vi "MAIN GENERA FILES STRINGHE.vi"(11 "This VI (main)":refnum<vi>) -> ()   [LabVIEW 2019]
uses:
  <vilib>/Utility/file.llb/Write Delimited Spreadsheet (string).vi
panel:
  out "Costanti":string[][](array[string])
  out "PageLabels":string[][](array[string])
  out "Strings[4]":string[][](array[string])
  out "Caption.Text":string[][](array[string])
  in  "target class 2":refnum<vi>
  in  "target class":refnum<vi>
  out "error out":errorcluster
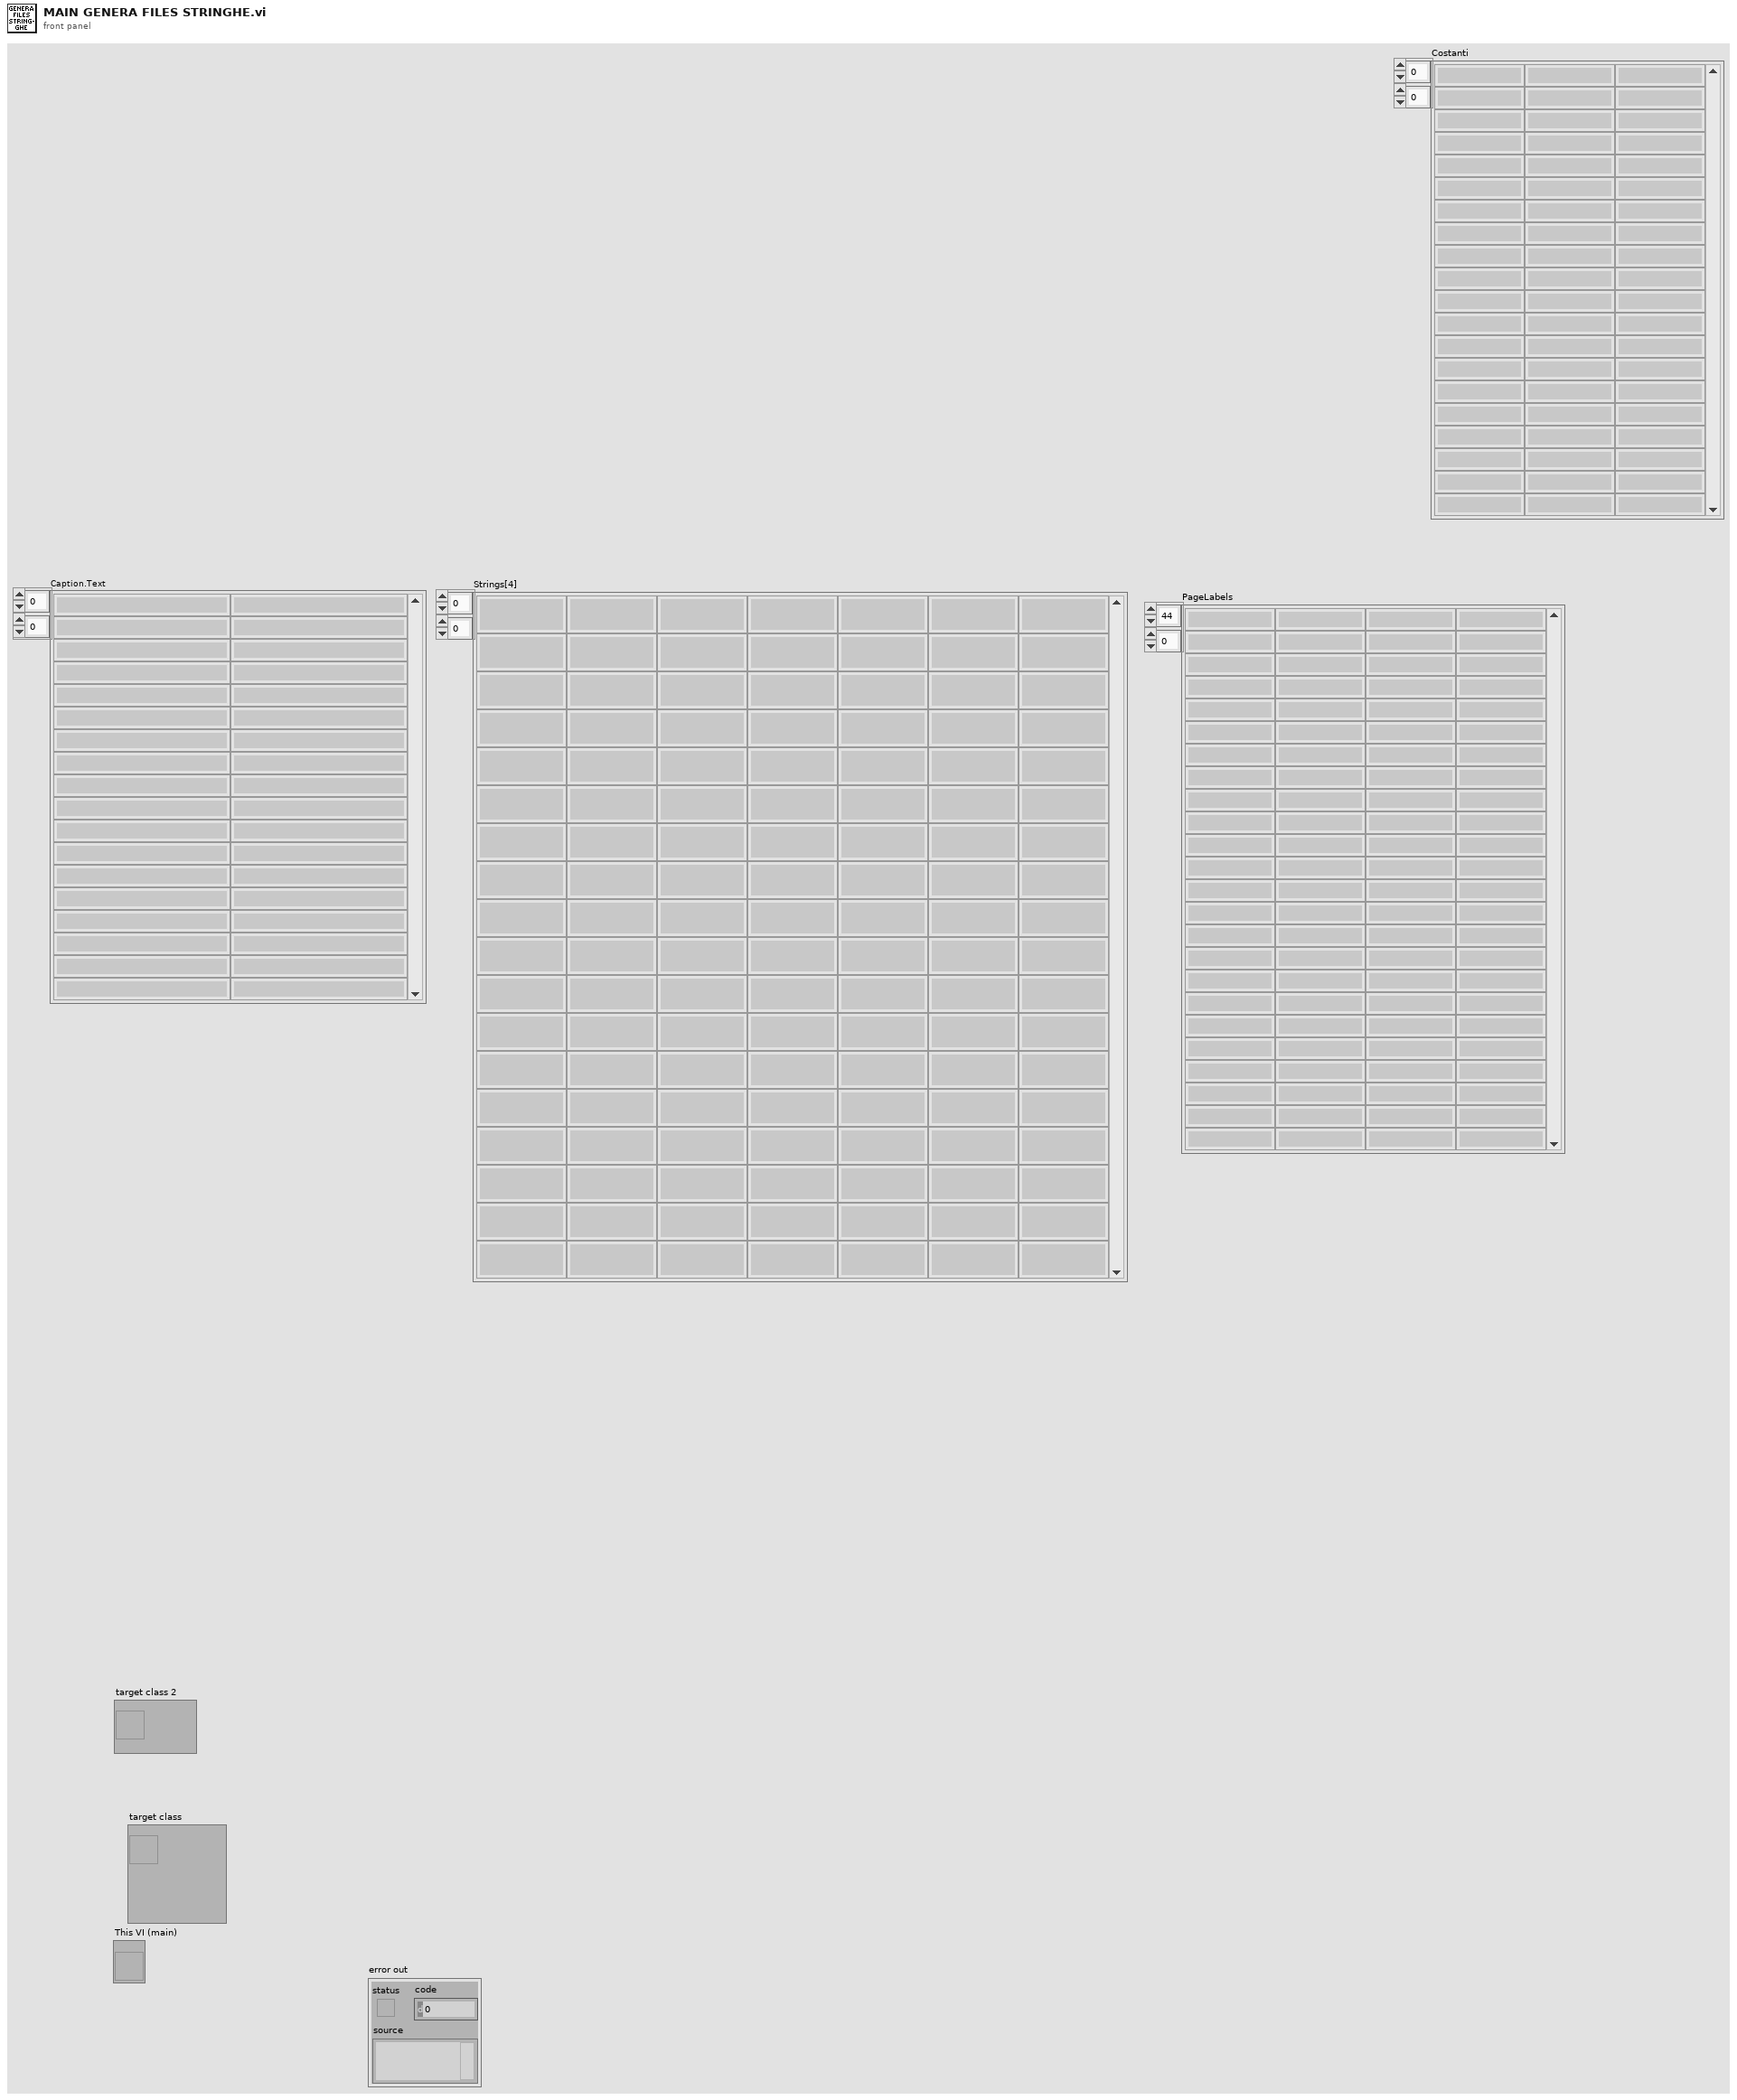
[diagram p1: front panel]
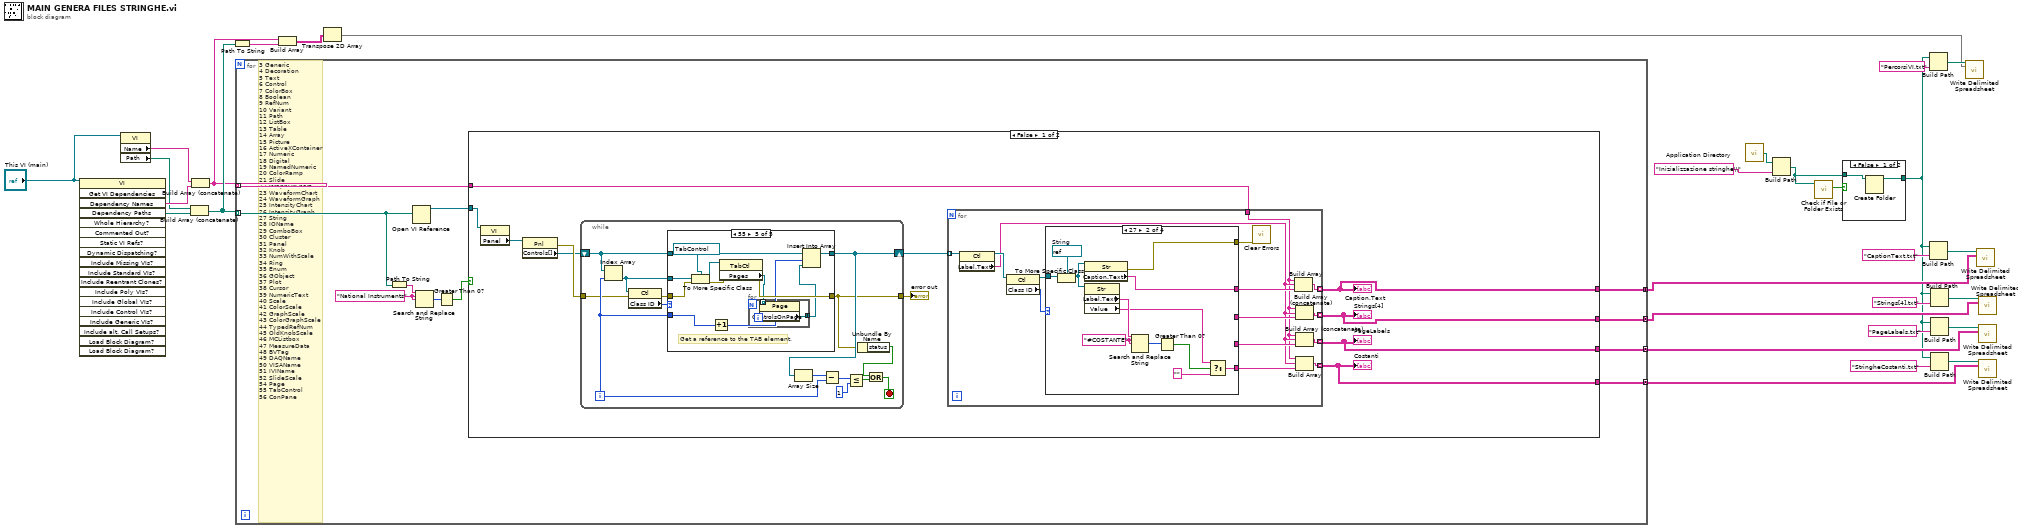
[diagram p0: block diagram]
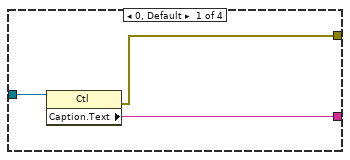
[diagram p3: hidden frame]
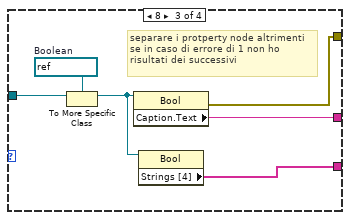
[diagram p4: hidden frame]
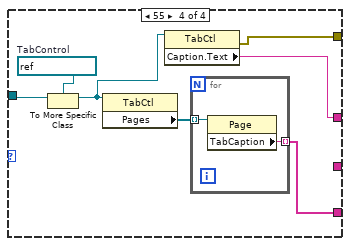
[diagram p5: hidden frame]
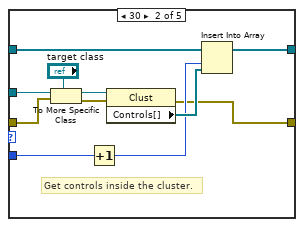
[diagram p7: hidden frame]
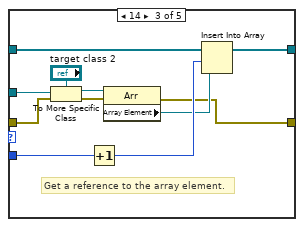
[diagram p8: hidden frame]
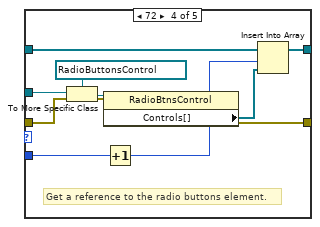
[diagram p9: hidden frame]
diagram:
  n1 = invoke class="VI" method="Get VI Dependencies"(reference="This VI (main)") -> ("Dependency Names"=w28:string[], "Dependency Paths"=w29:path[])  [unwired: 18 in, 17 out]
  n2 = property class="VI"(reference="This VI (main)") -> ("Name"=w27:string, "Path"=w26:path)  [unwired: 1 in, 2 out]
  n3 = Build Array (concatenate)(w26, w29) -> (w9:path[])
  n4 = Build Array (concatenate)(w27, w28) -> (w7:string[])
  n5 = Path To String(path=w9) -> (string=w8:string[])
  n6 = for {
    tunnel: w9 -> [w38] mode=indexing
    tunnel: w7 -> [w39] mode=indexing
    tunnel: [w33] -> w14 mode=concatenating
    tunnel: [w32] -> w13 mode=concatenating
    tunnel: [w31] -> w12 mode=concatenating
    tunnel: [w30] -> w11 mode=concatenating
    w36 = "National Instruments" ("search string")
    # "3\tGeneric\n4\tDecoration\n5\tText\n6\tControl\n7\tColorBox\n8\tBoolean\n9\tRefNum\n10\tVariant\n11\tPath\n12\tListBox\n13\tTable\n14\tArray\n15\tPicture\n16\tActiveXContainer\n17\tNumeric\n18\tDigital\n19\tNamedNumeric\n20\tColorRamp\n21\tSlide\n22\tGraphOrChart\n23\tWaveformChart\n24\tWaveformGraph\n25\tIntensityChart\n26\tIntensityGraph\n27\tString\n28\tIOName\n29\tComboBox\n30\tCluster\n31\tPanel\n32\tKnob\n33\tNumWithScale\n34\tRing\n35\tEnum\n36\tGObject\n37\tPlot\n38\tCursor\n39\tNumericText\n40\tScale\n41\tColorScale\n42\tGraphScale\n43\tColorGraphScale\n44\tTypedRefNum\n45\tOldKnobScale\n46\tMCListbox\n47\tMeasureData\n48\tBVTag\n49\tDAQName\n50\tVISAName\n51\tIVIName\n52\tSlideScale\n54\tPage\n55\tTabControl\n56\tConPane"
    n7 = Path To String(path=w38) -> (string=w37:string)
    n8 = Open VI Reference(vi path=w38) -> (vi reference=w40:refnum<vi>)  [unwired: 5 in, 1 out]
    n9 = Search and Replace String(input string=w37, search string=w36, replace string=w36) -> (number of replacements=w35:i32)  [unwired: 5 in, 3 out]
    n10 = Greater Than 0?(x=w35) -> (x > 0?=w34:bool)
    n11 = case shown="False" w34 {
      tunnel: w40 -> [w46 _]
      tunnel: w39 -> [w45 _]
      tunnel: [w41 _] -> w33
      tunnel: [w42 _] -> w32
      tunnel: [w43 _] -> w31
      tunnel: [w44 _] -> w30
      frame False {
        n12 = property class="VI"(reference=w46) -> ("Panel"=w48:refnum<vi>)  [unwired: 1 in, 2 out]
        n13 = property class="Pnl"(reference=w48) -> (error out=w50:errorcluster, "Controls[]"=w49:refnum<vi>[])  [unwired: 1 in, 1 out]
        n14 = while {
          shift-right: [w101] -> w47
          shift-left: w49 -> [w102]
          tunnel: w50 -> [w100]
          tunnel: [w97] -> w51
          i -> [w107]
          stop <- w105 stop-if-true
          n15 = Index Array(array=w102, index=w107) -> (element=w103:refnum<vi>)
          n16 = property class="Ctl"(reference=w103, error in=w100) -> (error out=w99:errorcluster, "Class ID"=w104:u32)  [unwired: 1 out]
          n17 = case shown="55" w104 {
            tunnel: w103 -> [_ w123 w134 w145 w157]
            tunnel: w102 -> [w112 w120 w131 w144 w156]
            tunnel: w107 -> [_ w119 w130 w143 w155]
            tunnel: [w112 w117 w129 w142 w154] -> w101
            tunnel: w99 -> [w111 w115 w126 w141 w153]
            tunnel: [w111 w113 w124 w140 w152] -> w97
            frame 0, Default {
            }
            frame 30 {
              # "Get controls inside the cluster."
              n18 = To More Specific Class(target class="target class", reference=w123, error in=w115) -> (specific class reference=w122:refnum<vi>, error out=w114:errorcluster)
              n19 = Increment(x=w119) -> (x+1=w116:i32)
              n20 = property class="Clust"(reference=w122, error in=w114) -> (error out=w113:errorcluster, "Controls[]"=w118:refnum<vi>[])  [unwired: 1 out]
              n21 = Insert Into Array(array=w120, index=w116, new element=w118) -> (w117:refnum<vi>[])
            }
            frame 14 {
              # "Get a reference to the array element."
              n22 = To More Specific Class(target class="target class 2", reference=w134, error in=w126) -> (specific class reference=w133:refnum<vi>, error out=w125:errorcluster)
              n23 = Increment(x=w130) -> (x+1=w128:i32)
              n24 = property class="Arr"(reference=w133, error in=w125) -> (error out=w124:errorcluster, "Array Element"=w127:refnum<vi>)  [unwired: 1 out]
              n25 = Insert Into Array(array=w131, index=w128, new element=w127) -> (w129:refnum<vi>[])
            }
            frame 72 {
              # "Get a reference to the radio buttons element."
              n26 = To More Specific Class(target class=refnum<vi> refnum ("Calcolo P2"), reference=w145, error in=w141) -> (specific class reference=w139:refnum<vi>, error out=w136:errorcluster)
              n27 = property class="RadioBtnsControl"(reference=w139, error in=w136) -> (error out=w140:errorcluster, "Controls[]"=w137:refnum<vi>[])  [unwired: 1 out]
              n28 = Increment(x=w143) -> (x+1=w138:i32)
              n29 = Insert Into Array(array=w144, index=w138, new element=w137) -> (w142:refnum<vi>[])
            }
            frame 55 {
              # "Get a reference to the TAB element."
              n30 = To More Specific Class(target class=refnum<vi> refnum ("Tab Control"), reference=w157, error in=w153) -> (specific class reference=w151:refnum<vi>, error out=w149:errorcluster)
              n31 = Increment(x=w155) -> (x+1=w150:i32)
              n32 = property class="TabCtl"(reference=w151, error in=w149) -> (error out=w152:errorcluster, "Pages"=w147:refnum<vi>[])  [unwired: 1 out]
              n33 = for {
                tunnel: w147 -> [w159] mode=indexing
                tunnel: [w158] -> w146 mode=concatenating
                n34 = property class="Page"(reference=w159) -> ("ControlsOnPage"=w158:refnum<vi>[])  [unwired: 1 in, 2 out]
              }
              n35 = Insert Into Array(array=w156, index=w150, new element=w146) -> (w154:refnum<vi>[])
            }
          }
          n36 = Array Size(array=w101) -> (size(s)=w110:i32)
          n37 = Subtract(x=w110, y=w107) -> (x-y=w109:i32)
          n38 = Less Or Equal?(x=w109, y=1) -> (x <= y?=w106:bool)
          n39 = Unbundle By Name(w97) -> ("status"=w98:bool)
          n40 = Or(x=w98, y=w106) -> (x .or. y?=w105:bool)
        }
        "error out" <- w51
        n41 = for {
          tunnel: w47 -> [w66] mode=indexing
          tunnel: [w61] -> w41 mode=indexing
          tunnel: [w59] -> w42 mode=indexing
          tunnel: [w56] -> w43 mode=indexing
          tunnel: [w54] -> w44 mode=indexing
          tunnel: w45 -> [w52]
          n42 = property class="Ctl"(reference=w66) -> (reference out=w58:refnum<vi>, "Label.Text"=w55:string)  [unwired: 1 in, 1 out]
          n43 = property class="Ctl"(reference=w58) -> (reference out=w64:refnum<vi>, "Class ID"=w65:u32)  [unwired: 1 in, 1 out]
          n44 = case shown="27" w65 {
            tunnel: w64 -> [w69 w77 w87 w94]
            tunnel: [w67 w72 w84 w89] -> w63
            tunnel: [_ _ w82 _] -> w60
            tunnel: [w68 w70 w85 w88] -> w62
            tunnel: [_ _ _ w91] -> w57
            tunnel: [_ w74 _ _] -> w53
            frame 0, Default {
              n45 = property class="Ctl"(reference=w69) -> (error out=w68:errorcluster, "Caption.Text"=w67:string)  [unwired: 1 in, 1 out]
            }
            frame 27 {
              w78 = refnum<vi> refnum  # String
              w80 = "#COSTANTE" ("search string")
              n46 = To More Specific Class(target class=w78, reference=w77) -> (specific class reference=w71:refnum<vi>)  [unwired: 1 in, 1 out]
              n47 = property class="Str"(reference=w71) -> (error out=w70:errorcluster, "Caption.Text"=w72:string)  [unwired: 1 in, 1 out]
              n48 = property class="Str"(reference=w71) -> ("Label.Text"=w81:string, "Value"=w75:string)  [unwired: 1 in, 2 out]
              n49 = Search and Replace String(input string=w81, search string=w80, replace string=w80) -> (number of replacements=w79:i32)  [unwired: 5 in, 3 out]
              n50 = Greater Than 0?(x=w79) -> (x > 0?=w76:bool)
              n51 = Select(t=w75, s=w76, f="") -> (s? t:f=w74:string)
            }
            frame 8 {
              w86 = refnum<vi> refnum  # Boolean
              # "separare i protperty node altrimenti\nse in caso di errore di 1 non ho \nrisultati dei successivi"
              n52 = To More Specific Class(target class=w86, reference=w87) -> (specific class reference=w83:refnum<vi>)  [unwired: 1 in, 1 out]
              n53 = property class="Bool"(reference=w83) -> (error out=w85:errorcluster, "Caption.Text"=w84:string)  [unwired: 1 in, 1 out]
              n54 = property class="Bool"(reference=w83) -> ("Strings [4]"=w82:string[])  [unwired: 1 in, 2 out]
            }
            frame 55 {
              w93 = refnum<vi> refnum  # TabControl
              n55 = To More Specific Class(target class=w93, reference=w94) -> (specific class reference=w90:refnum<vi>)  [unwired: 1 in, 1 out]
              n56 = property class="TabCtl"(reference=w90) -> ("Pages"=w92:refnum<vi>[])  [unwired: 1 in, 2 out]
              n57 = property class="TabCtl"(reference=w90) -> (error out=w88:errorcluster, "Caption.Text"=w89:string)  [unwired: 1 in, 1 out]
              n58 = for {
                tunnel: w92 -> [w96] mode=indexing
                tunnel: [w95] -> w91 mode=indexing
                n59 = property class="Page"(reference=w96) -> ("TabCaption"=w95:string)  [unwired: 1 in, 2 out]
              }
            }
          }
          n60 = call <vilib>:"Clear Errors.vi"("error in (no error)"=w62) -> ()  [unwired: 5 in, 2 out]
          n61 = Build Array(w52, w55, w63) -> (w61:string[])
          n62 = Build Array (concatenate)(w52, w55, w60) -> (w59:string[])
          n63 = Build Array (concatenate)(w52, w55, w57) -> (w56:string[])
          n64 = Build Array(w52, w55, w53) -> (w54:string[])
        }
        "Caption.Text" <- w41
        "Strings[4]" <- w42
        "PageLabels" <- w43
        "Costanti" <- w44
      }
      frame True {
        # "scarta i vi nella cartella national instruments (quelli della libreria labview)"
      }
    }
  }
  n65 = Build Array(w7, w8) -> (w6:string[][])
  n66 = Transpose 2D Array(2D array=w6) -> (transposed array=w3:string[][])
  n67 = call <vilib>:"Application Directory.vi"() -> ("Application Directory"=w15:path)
  n68 = Build Path(base path=w15, name or relative path="Inizializzazione stringhe\\") -> (appended path=w17:path)
  n69 = call <vilib>:"Check if File or Folder Exists.vi"("path"=w17) -> ("file or folder exists?"=w16:bool)  [unwired: 8 in, 2 out]
  n70 = case shown="False" w16 {
    tunnel: w17 -> [w161 w162]
    tunnel: [w160 w162] -> w5
    frame False {
      n71 = Create Folder(path (use dialog)=w161) -> (created path=w160:path)  [unwired: 2 in, 2 out]
    }
    frame True {
    }
  }
  n72 = Build Path(base path=w5, name or relative path="CaptionText.txt") -> (appended path=w18:path)
  n73 = Build Path(base path=w5, name or relative path="PercorsiVI.txt") -> (appended path=w4:path)
  n74 = Build Path(base path=w5, name or relative path="Strings[4].txt") -> (appended path=w23:path)
  n75 = Build Path(base path=w5, name or relative path="PageLabels.txt") -> (appended path=w21:path)
  n76 = Build Path(base path=w5, name or relative path="StringheCostanti.txt") -> (appended path=w25:path)
  n77 = call-poly <vilib>:"Write Delimited Spreadsheet.vi"("file path (dialog if empty)"=w4, "2D data"=w3) -> ()  [unwired: 12 in, 2 out]
  n78 = call-poly <vilib>:"Write Delimited Spreadsheet.vi"("file path (dialog if empty)"=w18, "2D data"=w14) -> ()  [unwired: 12 in, 2 out]
  n79 = call-poly <vilib>:"Write Delimited Spreadsheet.vi"("file path (dialog if empty)"=w23, "2D data"=w13) -> ()  [unwired: 12 in, 2 out]
  n80 = call-poly <vilib>:"Write Delimited Spreadsheet.vi"("file path (dialog if empty)"=w21, "2D data"=w12) -> ()  [unwired: 12 in, 2 out]
  n81 = call-poly <vilib>:"Write Delimited Spreadsheet.vi"("file path (dialog if empty)"=w25, "2D data"=w11) -> ()  [unwired: 12 in, 2 out]
